vi "Setup Maps and Queues.vi"(8 "error in (no error)":errorcluster, 11 "WAMP Client in":refnum<class "WAMP Client.lvclass">) -> (0 "error out":errorcluster, 3 "WAMP Client out":refnum<class "WAMP Client.lvclass">)   [LabVIEW 2021, in "wamplv.lvlib" / "WAMP Client.lvclass"]
uses:
  WAMP Client.lvclass
  WAMP Client.lvclass/WAMP Client.ctl
  TypeDef/EVENT payload.ctl
  API/TypeDefs/RESULT payload.ctl
  API/TypeDefs/WAMP error.ctl
  API/TypeDefs/Disconnected event data.ctl
  API/TypeDefs/INVOCATION payload.ctl
  TypeDef/Internal Message Type.ctl
  TypeDef/Internal Message.ctl
  TypeDef/Termination Reason Enum.ctl
  TypeDef/Termination Request.ctl
  TypeDef/Termination Reason.ctl
  API/TypeDefs/Combined error.ctl
  API/TypeDefs/Connected event data.ctl
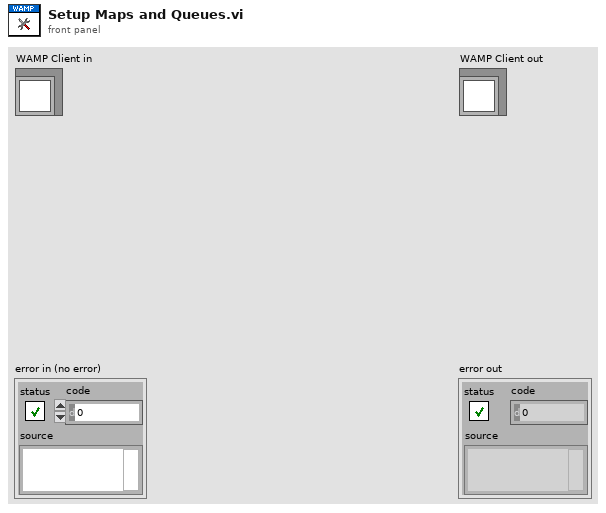
[diagram p1: front panel]
types:
  T1 = typedef "wamplv.lvlib/WAMP Client.lvclass/Connected event data.ctl" = cluster{"Session ID":u64}
  T2 = typedef "wamplv.lvlib/WAMP Client.lvclass/Disconnected event data.ctl" = cluster{"Error Out":errorcluster, "Termination Reason":T3}
  T3 = typedef "wamplv.lvlib/WAMP Client.lvclass/Termination Reason.ctl" = cluster{"Reason":T4, "Reason URI":string, "Message":string}
  T4 = typedef "wamplv.lvlib/WAMP Client.lvclass/Termination Reason Enum.ctl" = enum16{"Goodbye Received", "Abort Received", "Send Goodbye", "Send Abort", "Read Loop Failure", "Write Loop Failure", "Message Loop Failure"}
  T5 = typedef "wamplv.lvlib/WAMP Client.lvclass/Termination Request.ctl" = cluster{"Terminate?":bool, "Termination Reason":T3}
  T6 = typedef "wamplv.lvlib/WAMP Client.lvclass/Internal Message.ctl" = cluster{"Internal Message Type":T7, "Variant":variant}
  T7 = typedef "wamplv.lvlib/WAMP Client.lvclass/Internal Message Type.ctl" = enum16{"Subscribe", "Handle Subscribed", "Handle Event", "Unsubscribe", "Handle Unsubscribed", "Publish", "Handled Published", "Goodbye", "Handle Goodbye", "Call", "Handle Result", "Register", "Handle Registered", "Unregister", "Handle Unregistered", "Handle Invocation", "Yield", "Error"}
  T8 = typedef "wamplv.lvlib/WAMP Client.lvclass/EVENT payload.ctl" = cluster{"Arguments Payload":string, "ArgumentKw Payload":string, "Topic":string}
  T9 = typedef "wamplv.lvlib/WAMP Client.lvclass/INVOCATION payload.ctl" = cluster{"Arguments":string, "ArgumentKw":string, "Procedure URI":string, "Details":string, "Registration ID":u64, "Request ID":u64}
  T10 = typedef "wamplv.lvlib/WAMP Client.lvclass/RESULT payload.ctl" = cluster{"Arguments Payload":string, "ArgumentKw Payload":string, "Topic":string, "Combined Error":T11}
  T11 = typedef "wamplv.lvlib/WAMP Client.lvclass/Combined error.ctl" = cluster{"Error?":bool, "WAMP Error":T12, "Error":errorcluster}
  T12 = typedef "wamplv.lvlib/WAMP Client.lvclass/WAMP error.ctl" = cluster{"Details":string, "ArgumentKw Payload":string, "Error?":bool, "Error URI":string, "Arguments Payload":string}
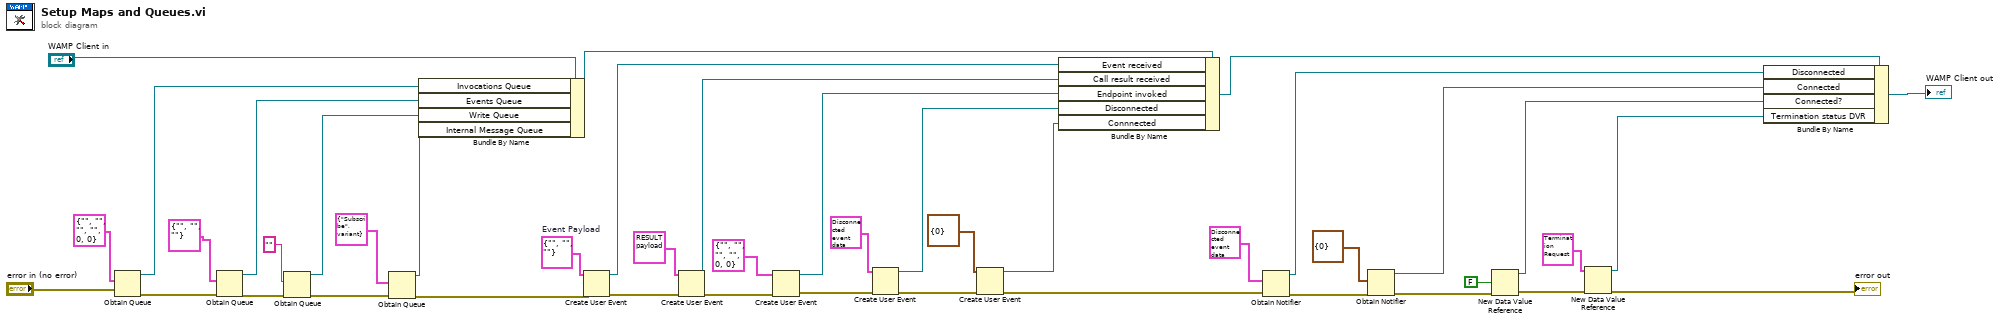
[diagram p0: block diagram]
diagram:
  w44 = T8 {"Arguments Payload"="", "ArgumentKw Payload"="", "Topic"=""}  # Event Payload
  n1 = Obtain Queue(element data type=T9 {"Arguments"="", "ArgumentKw"="", "Procedure URI"="", "Details"="", "Registration ID"=0, "Request ID"=0} ("INVOCATION payload"), error in (no error)="error in (no error)") -> (queue out=w26:refnum<queue>, error out=w35:errorcluster)  [unwired: 3 in, 1 out]
  n2 = Obtain Queue(element data type=T8 {"Arguments Payload"="", "ArgumentKw Payload"="", "Topic"=""} ("Cluster"), error in (no error)=w35) -> (queue out=w25:refnum<queue>, error out=w15:errorcluster)  [unwired: 3 in, 1 out]
  n3 = Obtain Queue(element data type="", error in (no error)=w15) -> (queue out=w18:refnum<queue>, error out=w16:errorcluster)  [unwired: 3 in, 1 out]
  n4 = Obtain Queue(element data type=T6 {"Internal Message Type"=enum."Subscribe", "Variant"=variant} ("Cluster"), error in (no error)=w16) -> (queue out=w17:refnum<queue>, error out=w2:errorcluster)  [unwired: 3 in, 1 out]
  n5 = Bundle By Name(cluster="WAMP Client in", "Invocations Queue"=w26, "Events Queue"=w25, "Write Queue"=w18, "Internal Message Queue"=w17) -> (w22:refnum<class "WAMP Client.lvclass">)
  n6 = Create User Event(user event datatype=w44, error in=w2) -> (user event=w21:refnum<user-event>, error out=w41:errorcluster)
  n7 = Create User Event(user event datatype=T10 {"Arguments Payload"="", "ArgumentKw Payload"="", "Topic"="", "Combined Error"={"Error?"=FALSE, "WAMP Error"={"Details"="{}", "ArgumentKw Payload"="", "Error?"=FALSE, "Error URI"="", "Arguments Payload"=""}, "Error"={"status"=FALSE, "code"=0, "source"=""}}} ("RESULT Payload"), error in=w41) -> (user event=w20:refnum<user-event>, error out=w38:errorcluster)
  n8 = Create User Event(user event datatype=T9 {"Arguments"="", "ArgumentKw"="", "Procedure URI"="", "Details"="", "Registration ID"=0, "Request ID"=0} ("INVOCATION payload"), error in=w38) -> (user event=w19:refnum<user-event>, error out=w8:errorcluster)
  n9 = Create User Event(user event datatype=T2 {"Error Out"={"status"=FALSE, "code"=0, "source"=""}, "Termination Reason"={"Reason"=enum."Goodbye Received", "Reason URI"="wamp.error.protocol_violation", "Message"=""}} ("Cluster"), error in=w8) -> (user event=w5:refnum<user-event>, error out=w6:errorcluster)
  n10 = Create User Event(user event datatype=T1 {"Session ID"=0} ("Connected event data"), error in=w6) -> (user event=w4:refnum<user-event>, error out=w3:errorcluster)
  n11 = Bundle By Name(cluster=w22, "Event received"=w21, "Call result received"=w20, "Endpoint invoked"=w19, "Disconnected"=w5, "Connnected"=w4) -> (w14:refnum<class "WAMP Client.lvclass">)
  n12 = Obtain Notifier(notification data type=T2 {"Error Out"={"status"=FALSE, "code"=0, "source"=""}, "Termination Reason"={"Reason"=enum."Goodbye Received", "Reason URI"="wamp.error.protocol_violation", "Message"=""}} ("Cluster"), error in (no error)=w3) -> (notifier out=w27:refnum<notifier>, error out=w12:errorcluster)  [unwired: 2 in, 1 out]
  n13 = Obtain Notifier(notification data type=T1 {"Session ID"=0} ("Connected event data"), error in (no error)=w12) -> (notifier out=w10:refnum<notifier>, error out=w13:errorcluster)  [unwired: 2 in, 1 out]
  n14 = New Data Value Reference(data value=FALSE, error in=w13) -> (data value reference=w31:refnum<data-value>, error out=w29:errorcluster)
  n15 = New Data Value Reference(data value=T5 {"Terminate?"=FALSE, "Termination Reason"={"Reason"=enum."Goodbye Received", "Reason URI"="wamp.error.protocol_violation", "Message"=""}} ("Daemon Termination Request"), error in=w29) -> (data value reference=w30:refnum<data-value>, error out=→"error out":errorcluster)
  n16 = Bundle By Name(cluster=w14, "Disconnected"=w27, "Connected"=w10, "Connected?"=w31, "Termination status DVR"=w30) -> (→"WAMP Client out":refnum<class "WAMP Client.lvclass">)
